vi "Display New Configuration SubPanel.vi"(8 "error in (no error)":errorcluster, 10 "ListBox Selection":i32, 11 "Configuration in":refnum<class "Configuration.lvclass">) -> (0 "error out":errorcluster, 3 "Configuration out":refnum<class "Configuration.lvclass">)   [LabVIEW 2016, in "Configuration.lvlib" / "Configuration.lvclass"]
uses:
  <userlib>/Configuration Dialog Actor/Configuration.lvclass
  <userlib>/Configuration Dialog Actor/Configuration.lvclass/Configuration.ctl
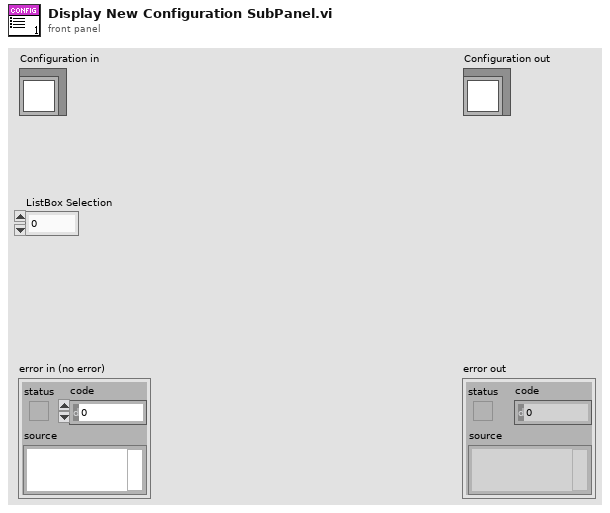
[diagram p1: front panel]
types:
  T1 = enum8{"Enabled", "Disabled", "Disabled and Grayed Out"}
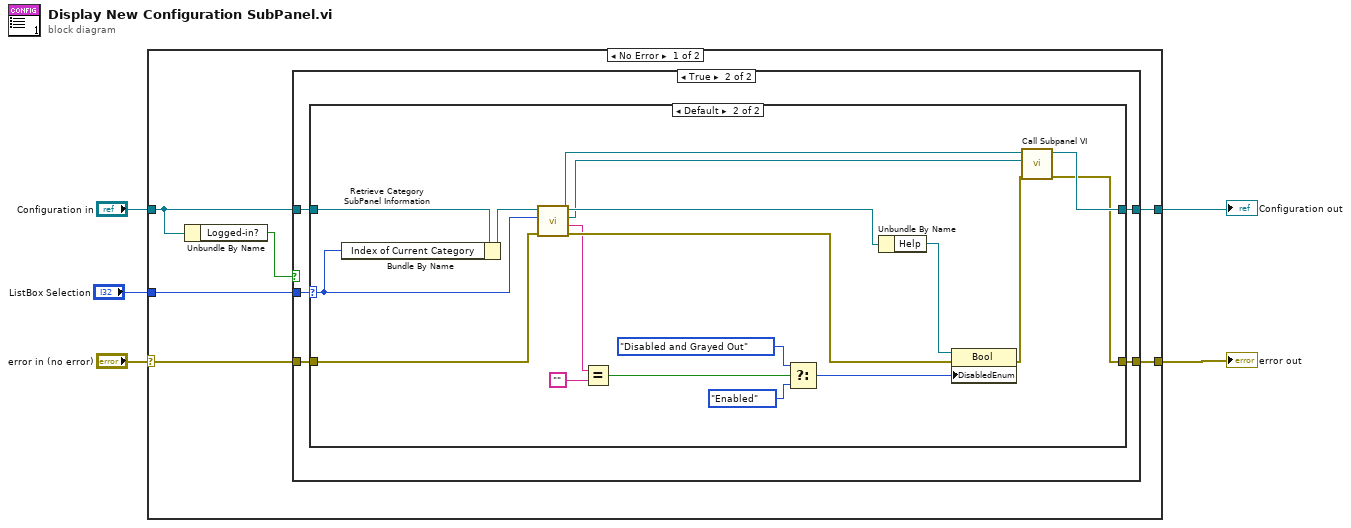
[diagram p0: block diagram]
diagram:
  n1 = case shown="No Error" "error in (no error)" {
    selector: "error in (no error)" -> [w10 w39]
    tunnel: [w9 w39] -> w4
    tunnel: [w11 w38] -> w2
    tunnel: "Configuration in" -> [w7 w38]
    tunnel: "ListBox Selection" -> [w8 _]
    frame No Error {
      n2 = Unbundle By Name(w7) -> ("Logged-in?"=w6:bool)
      n3 = case shown="True" w6 {
        tunnel: [w13 w18] -> w11
        tunnel: w10 -> [w12 w17]
        tunnel: [w12 w16] -> w9
        tunnel: w8 -> [_ w15]
        tunnel: w7 -> [w13 w14]
        frame False {
        }
        frame True {
          n4 = case shown="Default" w15 {
            selector: w15 -> [_ w25]
            tunnel: [w20 w37] -> w18
            tunnel: w17 -> [w19 w36]
            tunnel: [w19 w21] -> w16
            tunnel: w14 -> [w20 w35]
            frame -1 {
            }
            frame Default {
              n5 = Bundle By Name(cluster=w35, "Index of Current Category"=w25) -> (w24:refnum<class "Configuration.lvclass">)
              n6 = call <userlib>:"Retrieve Category SubPanel Information.vi"("error in (no error)"=w36, "ListBox Selection"=w25, "Configuration in"=w24) -> ("error out"=w27:errorcluster, "Help Text"=w23:string, "VI Refnum"=w22:refnum<vi>, "Configuration Out"=w26:refnum<class "Configuration.lvclass">)  [unwired: 5 in]
              n7 = Equal?(x=w23, y="") -> (x = y?=w31:bool)
              n8 = Select(t=T1."Disabled and Grayed Out" ("Disabled"), s=w31, f=T1."Enabled" ("Disabled")) -> (s? t:f=w30:T1)
              n9 = Unbundle By Name(w26) -> ("Help"=w33:refnum<vi>)
              n10 = property class="Bool"(reference=w33, error in=w27, "DisabledEnum"=w30) -> (error out=w32:errorcluster)  [unwired: 1 out]
              n11 = call-dynamic "Call Subpanel VI.vi"("error in (no error)"=w32, "VI Refnum"=w22, "Configuration in"=w26) -> ("error out"=w21:errorcluster, "Configuration out"=w37:refnum<class "Configuration.lvclass">)  [unwired: 7 in]
            }
          }
        }
      }
    }
    frame Error {
    }
  }
  "error out" <- w4
  "Configuration out" <- w2
